vi "Cycle K2450 Volt.vi"(1 "Action":T4=enum."Identify", 2 "Parameters":variant) -> (6 "Output":variant, 7 "Stop":bool)   [LabVIEW 2019]
doc: "This VI reads a single reading from a Keithley 2001 multimeter. The stop boolean is always false. If no reading is obtained a single zero is returned.\nScott Hannahs, NHMFL-FSU, Nov 1993"
uses:
  Sub Controls/Instrument Actions.ctl
  Sub Controls/Instrument Match.ctl
  Sub Controls/Public.ctl
  Sub Controls/Factory Reset.ctl
  Sub Controls/Scan Output.ctl
  Sub Controls/Instrument IDN.ctl
  Sub Controls/User Event Command.ctl
panel:
  in  "Factory Reset":T1
  in  "# Cycles":u32=5
  in  "Min Value":dbl=-20.0
  in  "Start Value":dbl
  in  "# Data Points at step":u32=2
  in  "Index":i32
  in  "Wait After Setting":dbl=3.0 format="%<%M:%S>t"
  in  "Max Value":dbl=20.0
  in  "Step Size":dbl=1.0 min=0.0
  out "Title":string
  in  "Public":T2
  in  "Address":u16(ring)
  out "Model":string
  in  "Instruments":T3[](array[typedef])=[{"Model"="MODEL 2450", "Manufacturer"="KEITHLEY INSTRUMENTS", "Term Character"="", "Wait Time (mS)"=0, "Wait for SRQ"=FALSE, "Type"="Voltage Source Cycle"}]
  out "Measurement":dbl[](array[numeric]) format="%^_7e"
  in  "VISA resource name":refnum<visa-resource-name>
  # "Term Char"
  # "Wait Time (mS)"
  # "Wait for SRQ?"
  # "Type"
  # "Manufacturer"
  # "Model"
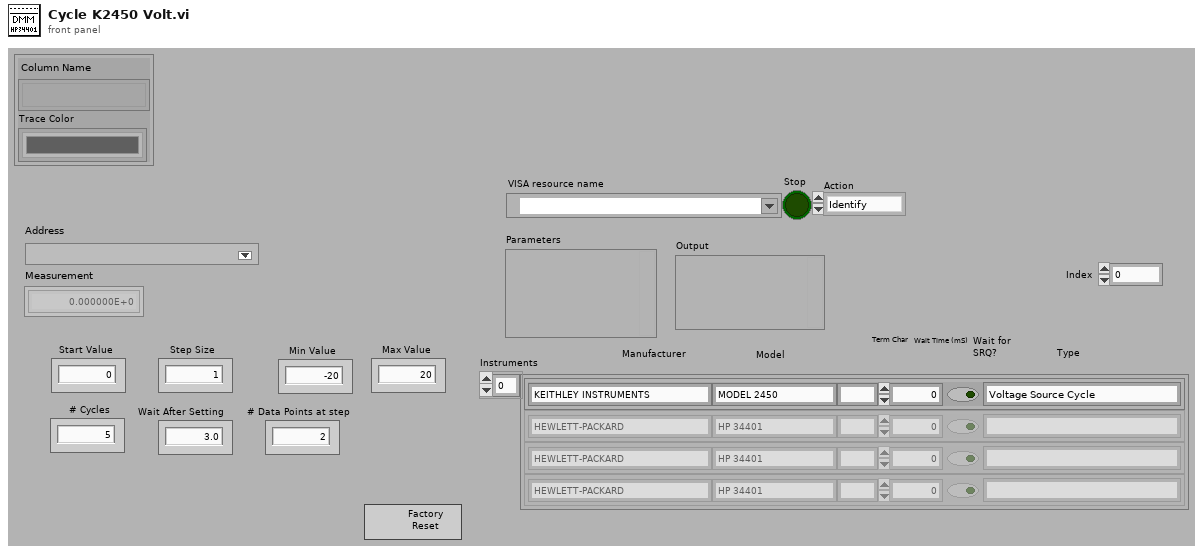
[diagram p1: front panel]
types:
  T1 = typedef "Factory Reset.ctl" = bool
  T2 = typedef "Public.ctl" = cluster{"Column Name":string[], "Trace Color":u32[]}
  T3 = typedef "Instrument Match.ctl" = cluster{"Model":string, "Manufacturer":string, "Term Character":string, "Wait Time (mS)":u32, "Wait for SRQ":bool, "Type":string}
  T4 = typedef "Instrument Actions.ctl" = enum16{"Scan", "Identify", "New", "Configure", "Initialize", "Test", "Read", "Close"}
  T5 = typedef "Scan Output.ctl" = cluster{"Manufacturer":string, "Model":string, "Info":string, "Revision":string, "error out":errorcluster}
  T6 = typedef "Instrument IDN.ctl" = cluster{"VISA Address":string, "Status":u16, "Manufacturer":string, "Model":string, "Info":string, "Info 2":string, "Misc Data":variant}
  T7 = typedef "User Event Command.ctl" = enum32{"Stop Config"}
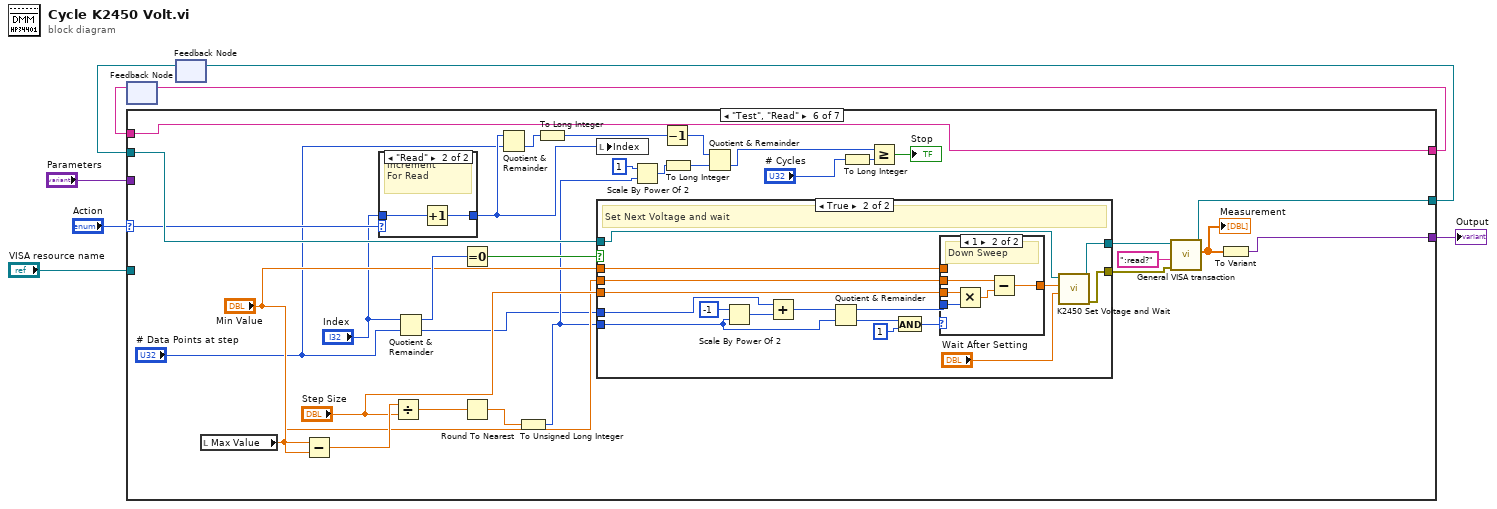
[diagram p0: block diagram]
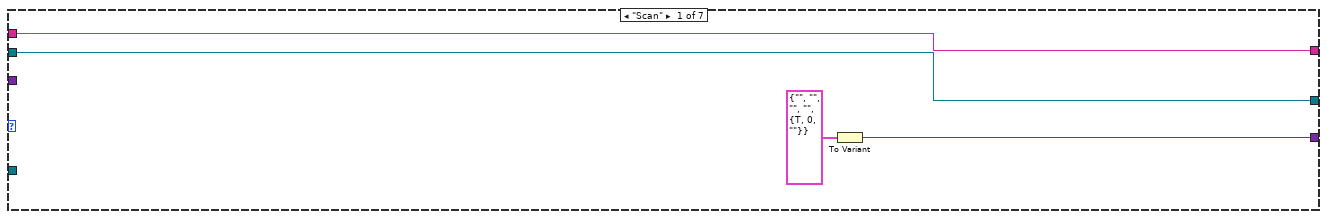
[diagram p2: hidden frame]
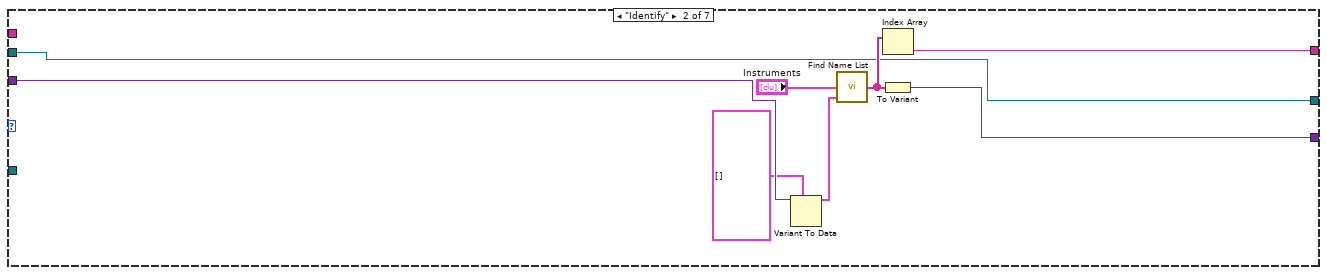
[diagram p3: hidden frame]
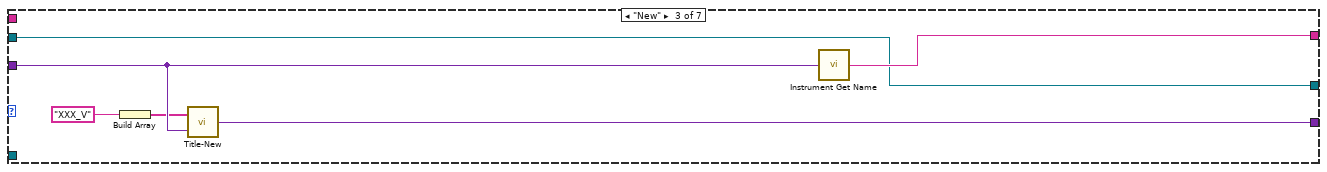
[diagram p4: hidden frame]
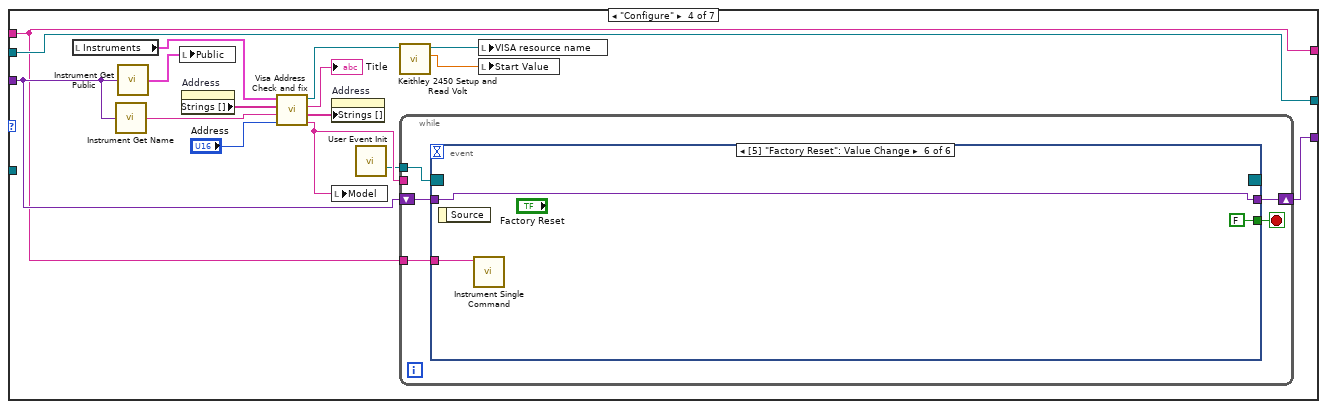
[diagram p5: hidden frame]
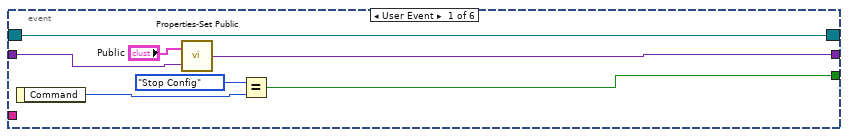
[diagram p6: hidden frame]
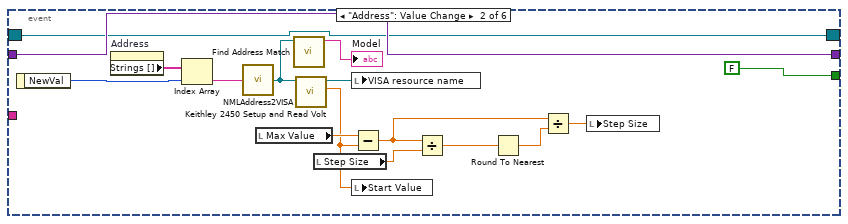
[diagram p7: hidden frame]
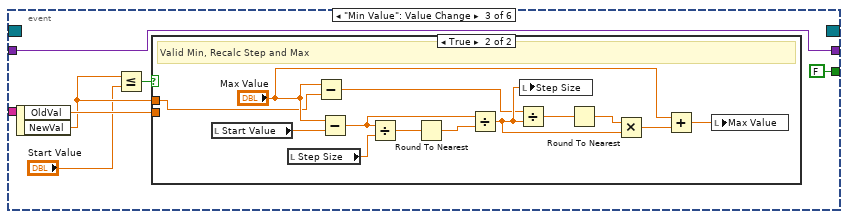
[diagram p8: hidden frame]
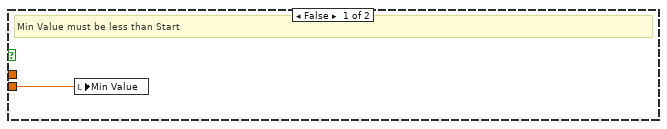
[diagram p9: hidden frame]
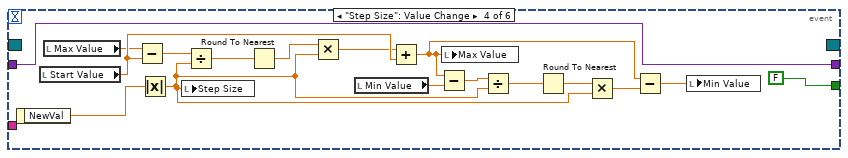
[diagram p10: hidden frame]
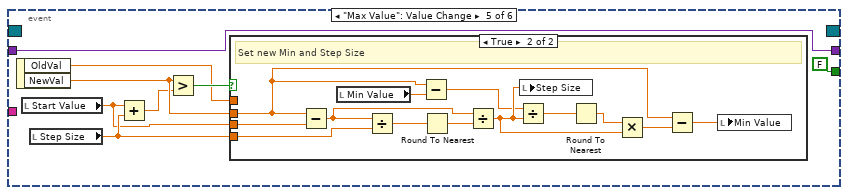
[diagram p11: hidden frame]
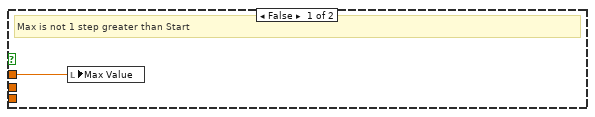
[diagram p12: hidden frame]
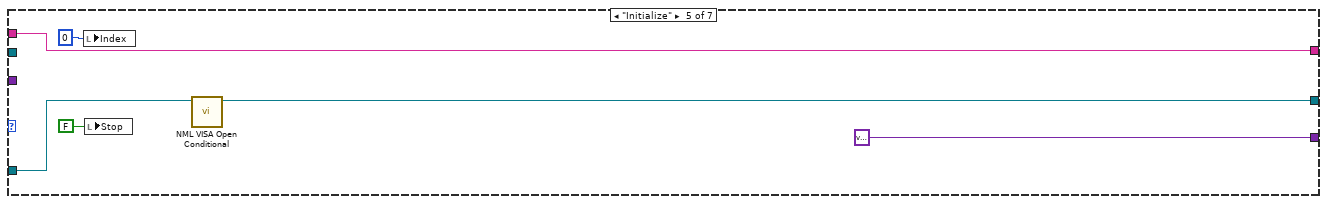
[diagram p13: hidden frame]
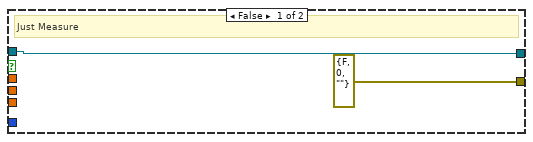
[diagram p14: hidden frame]
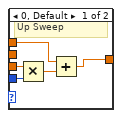
[diagram p15: hidden frame]
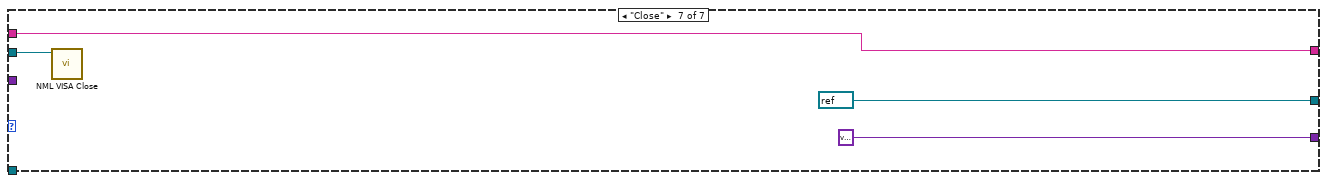
[diagram p17: hidden frame]
diagram:
  n1 = feedback #1() -> (w4:string)  [unwired: 1 in]
  n2 = feedback #2() -> (w1:refnum<visa-resource-name>)  [unwired: 1 in]
  n3 = case shown="\"Test\", \"Read\"" "Action" {
    selector: "Action" -> [_ _ _ _ _ w148 _]
    tunnel: [w12 w20 w26 w36 variant ("Variant") w170 variant ("Variant")] -> w7
    tunnel: "VISA resource name" -> [_ _ _ _ w138 _ _]
    tunnel: [w11 w15 w23 w27 w136 w168 w205] -> w5
    tunnel: w4 -> [w11 _ _ w27 w136 w168 w205]
    tunnel: "Parameters" -> [_ w19 w25 w34 _ _ _]
    tunnel: [w9 w13 w21 w29 w135 w169 refnum<visa-resource-name> refnum ("Open VISA Resource name")] -> w2
    tunnel: w1 -> [w9 w13 w21 w29 _ w165 w203]
    frame "Scan" {
      n4 = To Variant(anything=T5 {"Manufacturer"="", "Model"="", "Info"="", "Revision"="", "error out"={"status"=TRUE, "code"=0, "source"=""}} ("Scan Output")) -> (Variant=w12:variant)
    }
    frame "Identify" {
      n5 = Variant To Data(type=T6[] [], Variant=w19) -> (data=w17:T6[])  [unwired: 1 in, 1 out]
      n6 = call "Find Name List.vi"("Bus Scan"=w17, "Instruments"="Instruments") -> ("Names"=w14:string[])  [unwired: 1 in]
      n7 = Index Array(array=w14) -> (element=w15:string)  [unwired: 1 in]
      n8 = To Variant(anything=w14) -> (Variant=w20:variant)
    }
    frame "New" {
      n9 = Build Array("XXX_V") -> (w24:string[])
      n10 = call "Title-New.vi"("Parameters"=w25, "Array"=w24) -> ("Instrument Prop"=w26:variant)
      n11 = call "Instrument Get Name.vi"("Parameters"=w25) -> ("Type"=w23:string)
    }
    frame "Configure" {
      n12 = local read "Instruments"() -> (w39:T3[])
      n13 = call "Instrument Get Name.vi"("Parameters"=w34) -> ("Type"=w33:string)
      n14 = call "Instrument Get Public.vi"("Variant"=w34) -> ("Public"=w37:T2)
      n15 = local write "Public"(w37) -> ()
      n16 = property on="Address" class="Ring (strict)"() -> ("Strings []"=w40:string[])  [unwired: 2 in, 2 out]
      n17 = call "Visa Address Check and fix.vi"("Address"="Address", "Name"=w33, "NML Addresses"=w40, "Instruments"=w39) -> ("Model"=w38:string, "NML Addresses"=w42:string[], "Title"=→"Title":string, "VISA resource name"=w31:refnum<visa-resource-name>)  [unwired: 2 out]
      n18 = property on="Address" class="Ring (strict)"("Strings []"=w42) -> ()  [unwired: 2 in, 2 out]
      n19 = local write "Model"(w38) -> ()
      n20 = call "User Event Init.vi"() -> ("Event Registration Refnum"=w35:refnum<event-registration>)  [unwired: 14 in, 1 out]
      n21 = call "Keithley 2450 Setup and Read Volt.vi"("VISA Refnum in"=w31) -> ("Voltage"=w28:dbl, "VISA Refnum out"=w30:refnum<visa-resource-name>)  [unwired: 8 in, 1 out]
      n22 = while {
        tunnel: w38 -> [_]
        tunnel: w35 -> [w44]
        shift-right: [w47] -> w36
        shift-left: w34 -> [w45]
        tunnel: w27 -> [w43]
        stop <- w46 stop-if-true
        n23 = event shown="[5] \"Factory Reset\": Value Change" {
          selector: w44 -> [w48 w64 _ _ _ _]
          dyn-events: [w48 w64 _ _ _ _] -> _
          timeout: _ -> [_ _ _ _ _ _]
          tunnel: [w52 w65 w76 w107 w115 w131] -> w47
          tunnel: [w50 FALSE FALSE FALSE FALSE FALSE] -> w46
          tunnel: w45 -> [w53 w65 w76 w107 w115 w131]
          tunnel: w43 -> [_ _ _ _ _ w132]
          event User Event {
            n24 = event-data() -> ("Command"=w54:T7)  [unwired: 1 in]
            n25 = call "Properties-Set Public.vi"("Variant"=w53, "New Public"="Public") -> ("Variant 2"=w52:variant)
            n26 = Equal?(x=User_Event_Command."Stop Config", y=w54) -> (x = y?=w50:bool)
          }
          event "Address": Value Change {
            n27 = event-data() -> ("NewVal"=w70:u16)  [unwired: 1 in]
            n28 = property on="Address" class="Ring (strict)"() -> ("Strings []"=w67:string[])  [unwired: 2 in, 2 out]
            n29 = Index Array(array=w67, index=w70) -> (element=w68:string)
            n30 = call "NMLAddress2VISA.vi"("NML Address"=w68) -> ("VISA resource name"=w63:refnum<visa-resource-name>)
            n31 = local read "Max Value"() -> (w61:dbl)
            n32 = call "Find Address Match.vi"("VISA resource name"=w63) -> ("Model"=→"Model":string)  [unwired: 3 in, 3 out]
            n33 = call "Keithley 2450 Setup and Read Volt.vi"("VISA Refnum in"=w63) -> ("Voltage"=w59:dbl, "VISA Refnum out"=w62:refnum<visa-resource-name>)  [unwired: 8 in, 1 out]
            n34 = local read "Step Size"() -> (w58:dbl)
            n35 = local write "VISA resource name"(w62) -> ()
            n36 = local write "Start Value"(w59) -> ()
            n37 = Subtract(x=w61, y=w59) -> (x-y=w56:dbl)
            n38 = Divide(x=w56, y=w58) -> (x/y=w60:dbl)
            n39 = Round To Nearest(number=w60) -> (nearest integer value=w57:dbl)
            n40 = Divide(x=w56, y=w57) -> (x/y=w55:dbl)
            n41 = local write "Step Size"(w55) -> ()
          }
          event "Min Value": Value Change {
            n42 = event-data() -> ("OldVal"=w74:dbl, "NewVal"=w73:dbl)  [unwired: 1 in]
            n43 = Less Or Equal?(x=w73, y="Start Value") -> (x <= y?=w75:bool)
            n44 = case shown="True" w75 {
              tunnel: w74 -> [w77 _]
              tunnel: w73 -> [_ w78]
              frame False {
                # "Min Value must be less than Start"
                n45 = local write "Min Value"(w77) -> ()
              }
              frame True {
                # "Valid Min, Recalc Step and Max"
                n46 = local read "Start Value"() -> (w80:dbl)
                n47 = local read "Step Size"() -> (w88:dbl)
                n48 = Subtract(x="Max Value", y=w78) -> (x-y=w81:dbl)
                n49 = Subtract(x="Max Value", y=w80) -> (x-y=w87:dbl)
                n50 = Divide(x=w87, y=w88) -> (x/y=w79:dbl)
                n51 = Round To Nearest(number=w79) -> (nearest integer value=w86:dbl)
                n52 = Divide(x=w87, y=w86) -> (x/y=w89:dbl)
                n53 = Divide(x=w81, y=w89) -> (x/y=w82:dbl)
                n54 = local write "Step Size"(w89) -> ()
                n55 = Round To Nearest(number=w82) -> (nearest integer value=w83:dbl)
                n56 = Multiply(x=w83, y=w89) -> (x*y=w85:dbl)
                n57 = Add(x="Max Value", y=w85) -> (x+y=w84:dbl)
                n58 = local write "Max Value"(w84) -> ()
              }
            }
          }
          event "Step Size": Value Change {
            n59 = event-data() -> ("NewVal"=w106:dbl)  [unwired: 1 in]
            n60 = local read "Start Value"() -> (w98:dbl)
            n61 = local read "Max Value"() -> (w93:dbl)
            n62 = Subtract(x=w93, y=w98) -> (x-y=w94:dbl)
            n63 = Absolute Value(x=w106) -> (abs(x)=w92:dbl)
            n64 = local write "Step Size"(w92) -> ()
            n65 = Divide(x=w94, y=w92) -> (x/y=w95:dbl)
            n66 = Round To Nearest(number=w95) -> (nearest integer value=w96:dbl)
            n67 = Multiply(x=w96, y=w92) -> (x*y=w97:dbl)
            n68 = local read "Min Value"() -> (w99:dbl)
            n69 = Add(x=w97, y=w98) -> (x+y=w103:dbl)
            n70 = Subtract(x=w103, y=w99) -> (x-y=w100:dbl)
            n71 = local write "Max Value"(w103) -> ()
            n72 = Divide(x=w100, y=w92) -> (x/y=w101:dbl)
            n73 = Round To Nearest(number=w101) -> (nearest integer value=w102:dbl)
            n74 = Multiply(x=w102, y=w92) -> (x*y=w105:dbl)
            n75 = Subtract(x=w103, y=w105) -> (x-y=w104:dbl)
            n76 = local write "Min Value"(w104) -> ()
          }
          event "Max Value": Value Change {
            n77 = event-data() -> ("OldVal"=w109:dbl, "NewVal"=w114:dbl)  [unwired: 1 in]
            n78 = local read "Start Value"() -> (w112:dbl)
            n79 = local read "Step Size"() -> (w113:dbl)
            n80 = Add(x=w112, y=w113) -> (x+y=w111:dbl)
            n81 = Greater?(x=w114, y=w111) -> (0:w110:bool)
            n82 = case shown="True" w110 {
              tunnel: w114 -> [_ w119]
              tunnel: w113 -> [_ w118]
              tunnel: w112 -> [_ w117]
              tunnel: w109 -> [w116 _]
              frame False {
                # "Max is not 1 step greater than Start"
                n83 = local write "Max Value"(w116) -> ()
              }
              frame True {
                # "Set new Min and Step Size"
                n84 = Subtract(x=w119, y=w117) -> (x-y=w128:dbl)
                n85 = local read "Min Value"() -> (w121:dbl)
                n86 = Divide(x=w128, y=w118) -> (x/y=w120:dbl)
                n87 = Subtract(x=w119, y=w121) -> (x-y=w122:dbl)
                n88 = Round To Nearest(number=w120) -> (nearest integer value=w127:dbl)
                n89 = Divide(x=w128, y=w127) -> (x/y=w129:dbl)
                n90 = Divide(x=w122, y=w129) -> (x/y=w123:dbl)
                n91 = local write "Step Size"(w129) -> ()
                n92 = Round To Nearest(number=w123) -> (nearest integer value=w124:dbl)
                n93 = Multiply(x=w124, y=w129) -> (x*y=w126:dbl)
                n94 = Subtract(x=w119, y=w126) -> (x-y=w125:dbl)
                n95 = local write "Min Value"(w125) -> ()
              }
            }
          }
          event Value Change {
            n96 = event-data() -> ()  [unwired: 1 in, 1 out]
            n97 = call "Instrument Single Command.vi"("VISA Name"=w132) -> ()  [unwired: 10 in, 1 out]
          }
        }
      }
      n98 = local write "VISA resource name"(w30) -> ()
      n99 = local write "Start Value"(w28) -> ()
    }
    frame "Initialize" {
      n100 = local write "Index"(0 ("Index")) -> ()
      n101 = local write "Stop"(FALSE ("Stop")) -> ()
      n102 = call "NML VISA Open Conditional.vi"("VISA resource name"=w138) -> ("dup VISA Session"=w135:refnum<visa-resource-name>)  [unwired: 8 in, 2 out]
    }
    frame "Test", "Read" {
      n103 = local read "Max Value"() -> (w150:dbl)
      n104 = Subtract(x=w150, y="Min Value") -> (x-y=w153:dbl)
      n105 = case shown="\"Read\"" w148 {
        tunnel: "Index" -> [w200 w202]
        tunnel: [w200 w201] -> w144
        frame "Test", Default {
          # "Leave\nfor Test"
        }
        frame "Read" {
          # "Increment \nFor Read"
          n106 = Increment(x=w202) -> (x+1=w201:i32)
        }
      }
      n107 = Divide(x=w153, y="Step Size") -> (x/y=w154:dbl)
      n108 = Quotient & Remainder(x="Index", y="# Data Points at step") -> (x-y*floor(x/y)=w167:u32, floor(x/y)=w146:u32)
      n109 = Equal To 0?(x=w167) -> (x = 0?=w166:bool)
      n110 = Round To Nearest(number=w154) -> (nearest integer value=w155:dbl)
      n111 = Quotient & Remainder(x=w144, y="# Data Points at step") -> (floor(x/y)=w145:u32)  [unwired: 1 out]
      n112 = To Unsigned Long Integer(number=w155) -> (unsigned 32bit integer=w149:u32)
      n113 = To Long Integer(number=w145) -> (32bit integer=w141:i32)
      n114 = local write "Index"(w144) -> ()
      n115 = case shown="True" w166 {
        tunnel: w146 -> [_ w177]
        tunnel: w165 -> [w172 w189]
        tunnel: [w172 w188] -> w164
        tunnel: [errorcluster {"status"=FALSE, "code"=0, "source"=""} ("error out") w187] -> w161
        tunnel: w149 -> [_ w176]
        tunnel: "Step Size" -> [_ w175]
        tunnel: "Min Value" -> [_ w174]
        tunnel: w150 -> [_ w173]
        frame False {
          # "Just Measure"
        }
        frame True {
          # "Set Next Voltage and wait"
          n116 = Scale By Power Of 2(n=i16 -1, x=w176) -> (x*2^n=w182:u32)
          n117 = Add(x=w177, y=w182) -> (x+y=w183:u32)
          n118 = Quotient & Remainder(x=w183, y=w176) -> (x-y*floor(x/y)=w186:u32, floor(x/y)=w184:u32)
          n119 = And(x=w184, y=u32 1) -> (x .and. y?=w185:u32)
          n120 = case shown="1" w185 {
            tunnel: w174 -> [w194 _]
            tunnel: w186 -> [w193 w199]
            tunnel: w175 -> [w191 w197]
            tunnel: [w190 w196] -> w178
            tunnel: w173 -> [_ w195]
            frame 0, Default {
              # "Up Sweep"
              n121 = Multiply(x=w191, y=w193) -> (x*y=w192:dbl)
              n122 = Add(x=w194, y=w192) -> (x+y=w190:dbl)
            }
            frame 1 {
              # "Down Sweep"
              n123 = Multiply(x=w197, y=w199) -> (x*y=w198:dbl)
              n124 = Subtract(x=w195, y=w198) -> (x-y=w196:dbl)
            }
          }
          n125 = call "K2450 Set Voltage and Wait.vi"("Wait After Setting"="Wait After Setting", "Voltage"=w178, "VISA resource name"=w189) -> ("Error Out"=w187:errorcluster, "VISA resource name Out"=w188:refnum<visa-resource-name>)  [unwired: 7 in]
        }
      }
      n126 = Scale By Power Of 2(n=i16 1, x=w149) -> (x*2^n=w157:u32)
      n127 = Decrement(x=w141) -> (x-1=w142:i32)
      n128 = To Long Integer(number=w157) -> (32bit integer=w140:i32)
      n129 = Quotient & Remainder(x=w142, y=w140) -> (floor(x/y)=w159:i32)  [unwired: 1 out]
      n130 = To Long Integer(number="# Cycles") -> (32bit integer=w139:i32)
      n131 = Greater Or Equal?(x=w159, y=w139) -> (x >= y?=→"Stop":bool)
      n132 = call "General VISA transaction.vi"("error in (no error)"=w161, "Command String"=":read?", "VISA Session"=w164) -> ("Measurement"=w162:dbl[], "dup VISA Session"=w169:refnum<visa-resource-name>)  [unwired: 3 in, 4 out]
      "Measurement" <- w162
      n133 = To Variant(anything=w162) -> (Variant=w170:variant)
    }
    frame "Close" {
      n134 = call "NML VISA Close.vi"("VISA resource name"=w203) -> ()  [unwired: 10 in, 1 out]
    }
  }
  "Output" <- w7
  n135 = feedback-in #1(w5) -> ()
  n136 = feedback-in #2(w2) -> ()
